vi "Get Bucket RequestPayment Configuration.vi"(8 "error in (no error)":errorcluster, 9 "Bucket":string) -> (0 "error out":errorcluster, 3 "RequestPaymentConfiguration":T1)   [LabVIEW 2011, in "LV Interface for Amazon S3.lvlib"]
doc: "This operation <B>returns the request payment configuration</B> of a bucket. To use this version of the operation, <B>you must be the bucket owner</B>."
uses:
  LV Interface for Amazon S3.lvlib
  Typedefs/AMZ_S3_API_RequestPaymentConfig.ctl
  Typedefs/AMZ_S3_Payer.ctl
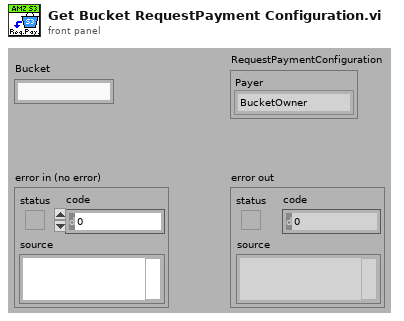
[diagram p1: front panel]
types:
  T1 = typedef "LV Interface for Amazon S3.lvlib/AMZ_S3_API_RequestPaymentConfig.ctl" = cluster{"Payer":T2}
  T2 = typedef "LV Interface for Amazon S3.lvlib/AMZ_S3_Payer.ctl" = enum16{"BucketOwner", "Requester"}
  T3 = typedef "LV Interface for Amazon S3.lvlib/AMZ_S3_Call Results.ctl" = enum16{"Success", "UndefinedError", "AccessDenied", "AccountProblem", "AmbiguousGrantByEmailAddress", "BadDigest", "BucketAlreadyExists", "BucketAlreadyOwnedByYou", "BucketNotEmpty", "CredentialsNotSupported", "CrossLocationLoggingProhibited", "EntityTooSmall", "EntityTooLarge", "ExpiredToken", "IllegalVersioningConfigurationException", "IncompleteBody", "IncorrectNumberOfFilesInPostRequest", "InlineDataTooLarge", "InternalError", "InvalidAccessKeyId", "InvalidAddressingHeader", "InvalidArgument", "InvalidBucketName", "InvalidDigest", "InvalidLocationConstraint", "InvalidPart", "InvalidPartOrder", "InvalidPayer", "InvalidPolicyDocument", "InvalidRange", "InvalidSecurity", "InvalidSOAPRequest", "InvalidStorageClass", "InvalidTargetBucketForLogging", "InvalidToken", "InvalidURI", "KeyTooLong", "MalformedACLError", "MalformedPOSTRequest", "MalformedXML", "MaxMessageLengthExceeded", "MaxPostPreDataLengthExceededError", "MetadataTooLarge", "MethodNotAllowed", "MissingAttachment", "MissingContentLength", "MissingRequestBodyError", "MissingSecurityElement", "MissingSecurityHeader", "NoLoggingStatusForKey", "NoSuchBucket", "NoSuchKey", "NoSuchUpload", "NoSuchVersion", "NotImplemented", "NotSignedUp", "OperationAborted", "PermanentRedirect", "PreconditionFailed", "Redirect", "RequestIsNotMultiPartContent", "RequestTimeout", "RequestTimeTooSkewed", "RequestTorrentOfBucketError", "SignatureDoesNotMatch", "SlowDown", "TemporaryRedirect", "TokenRefreshRequired", "TooManyBuckets", "UnexpectedContent", "UnresolvableGrantByEmailAddress", "UserKeyMustBeSpecified", "LabVIEWError"}
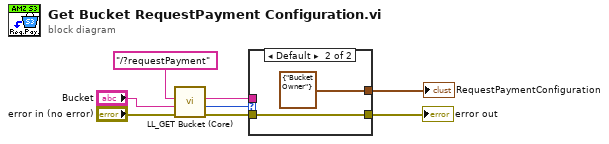
[diagram p0: block diagram]
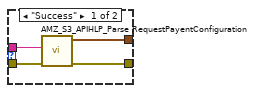
[diagram p2: hidden frame]
diagram:
  n1 = call "LL_GET Bucket (Core).vi"("error in (no error)"="error in (no error)", "Bucket"="Bucket", "Path and query string"="/?requestPayment") -> ("error out"=w4:errorcluster, "Call Result"=w5:T3, "Response body"=w3:string)  [unwired: 5 in, 1 out]
  n2 = case shown="Default" w5 {
    tunnel: w4 -> [w12 w13]
    tunnel: w3 -> [w11 _]
    tunnel: [w10 w13] -> w2
    tunnel: [w9 T1 {"Payer"=enum."BucketOwner"} ("RequestPaymentConfiguration")] -> w1
    frame "Success" {
      n3 = call "AMZ_S3_APIHLP_Parse RequestPayentConfiguration.vi"("error in (no error)"=w12, "Response body"=w11) -> ("error out"=w10:errorcluster, "RequestPaymentConfiguration"=w9:T1)  [unwired: 8 in]
    }
    frame Default {
    }
  }
  "error out" <- w2
  "RequestPaymentConfiguration" <- w1
